vi "Write Source Waveform.vi"(0 "RFFE Command in":refnum<class "RFFE Command.lvclass">, 5 "instrument handle":refnum<k15>, 7 "Waveform Data":u32[](array[numeric]) format="%.0x", 11 "error in (no error)":errorcluster) -> (4 "RFFE Command out":refnum<class "RFFE Command.lvclass">, 6 "instrument handle out":refnum<k15>, 15 "error out":errorcluster)   [LabVIEW 2018, in "MIPI RFFE API.lvlib" / "RFFE Command.lvclass"]
uses:
  RFFE Command.lvclass
  <instrlib>/niDigital/niDigital.llb/niDigital Write Source Waveform (Broadcast U32).vi
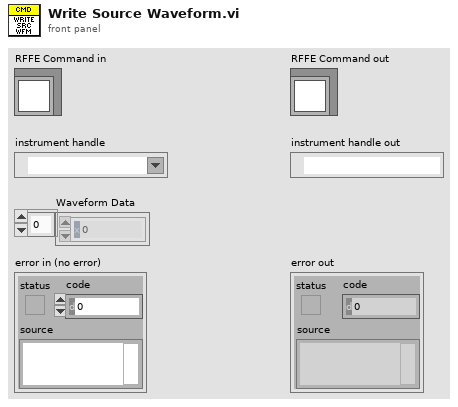
[diagram p1: front panel]
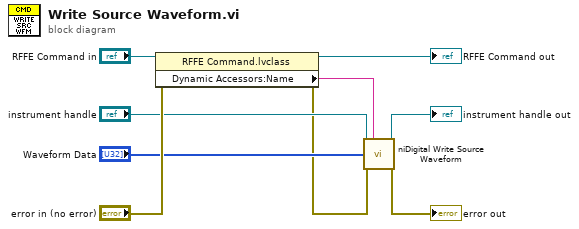
[diagram p0: block diagram]
diagram:
  n1 = property class="RFFE Command.lvclass"(reference="RFFE Command in", error in="error in (no error)") -> (reference out=→"RFFE Command out":refnum<class "RFFE Command.lvclass">, error out=w1:errorcluster, "Dynamic Accessors:Name"=w2:string)
  n2 = call-poly <instrlib>:"niDigital Write Source Waveform.vi"("instrument handle"="instrument handle", "waveform name"=w2, "waveform data"="Waveform Data", "error in"=w1) -> ("instrument handle out"=→"instrument handle out":refnum<k15>, "error out"=→"error out":errorcluster)  [unwired: 10 in]
